vi "Voltage Display.vi"(0 "RedPitaya connection in":refnum<k5>, 2 "Vertical Offset":dbl, 3 "Vertical Scale":dbl, 5 "error in":errorcluster, 8 "Channel #":u16(ring) items=["Channel 1", "Channel 2"], 12 "timeout ms (2000)":i32) -> (14 "RedPitaya connection out":refnum<k5>, 19 "error out":errorcluster)   [LabVIEW 8.6]
doc: "Sets vertical offset and scale of selected channel"
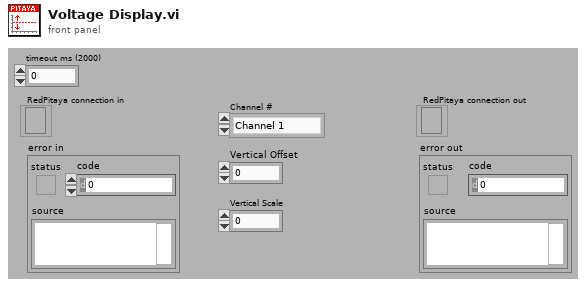
[diagram p1: front panel]
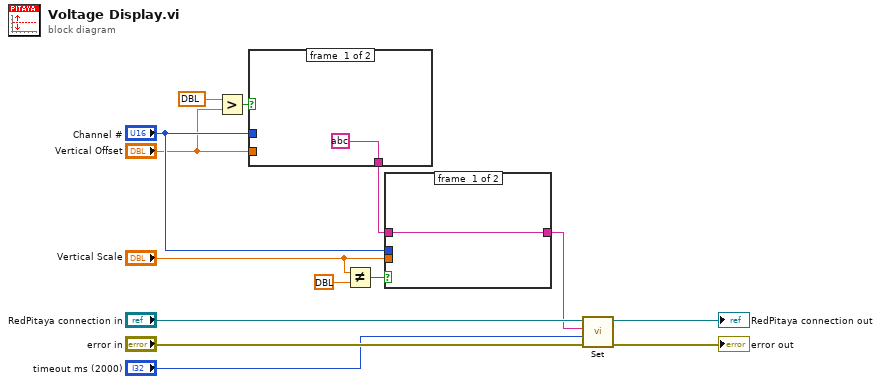
[diagram p0: block diagram]
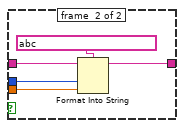
[diagram p2: hidden frame]
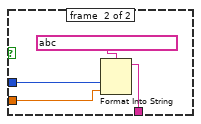
[diagram p3: hidden frame]
diagram:
  n1 = Greater?(x=dbl ?, y="Vertical Offset") -> (0:w7:bool)
  n2 = case shown="True" w7 {
    tunnel: "Vertical Offset" -> [_ w18]
    tunnel: [string ? w17] -> w10
    tunnel: "Channel #" -> [_ w16]
    frame #0 {
    }
    frame #1 {
      n3 = Format Into String(format string=string ?, w16, w18) -> (resulting string=w17:string)  [unwired: 2 in, 1 out]
    }
  }
  n4 = Not Equal?(x="Vertical Scale", y=dbl ?) -> (x != y?=w4:bool)
  n5 = case shown="True" w4 {
    tunnel: w10 -> [w20 w25]
    tunnel: "Channel #" -> [_ w23]
    tunnel: "Vertical Scale" -> [_ w22]
    tunnel: [w20 w21] -> w8
    frame #0 {
    }
    frame #1 {
      n6 = Format Into String(format string=string ?, initial string=w25, w23, w22) -> (resulting string=w21:string)  [unwired: 1 in, 1 out]
    }
  }
  n7 = call "Set.vi"("error in"="error in", "timeout ms (2000)"="timeout ms (2000)", "SCPI Message"=w8, "RedPitaya connection in"="RedPitaya connection in") -> ("error out"=→"error out":errorcluster, "RedPitaya connection out"=→"RedPitaya connection out":refnum<k5>)  [unwired: 5 in, 1 out]
